vi "depth threshold test.vi"(1 "Depth\nPrevious":dbl format="%.2f", 2 "Depth \nCurrent":dbl format="%.2f") -> (0 "Threshold\nExceeded":bool)   [LabVIEW 2016]
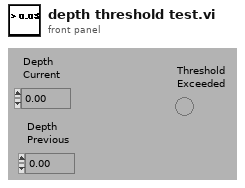
[diagram p1: front panel]
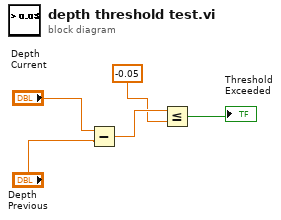
[diagram p0: block diagram]
diagram:
  n1 = Subtract(x="Depth \nCurrent", y="Depth\nPrevious") -> (x-y=w3:dbl)
  n2 = Less Or Equal?(x=w3, y=-0.05) -> (x <= y?=→"Threshold\nExceeded":bool)
